vi "deleteBlankData.vi"(8 "error in (no error)":errorcluster, 11 "reference in":refnum<class "Notification Controller.lvclass">) -> (0 "error out":errorcluster, 3 "reference out":refnum<class "Notification Controller.lvclass">)   [LabVIEW 2015, in "Notification Controller.lvclass"]
uses:
  Notification Controller.lvclass
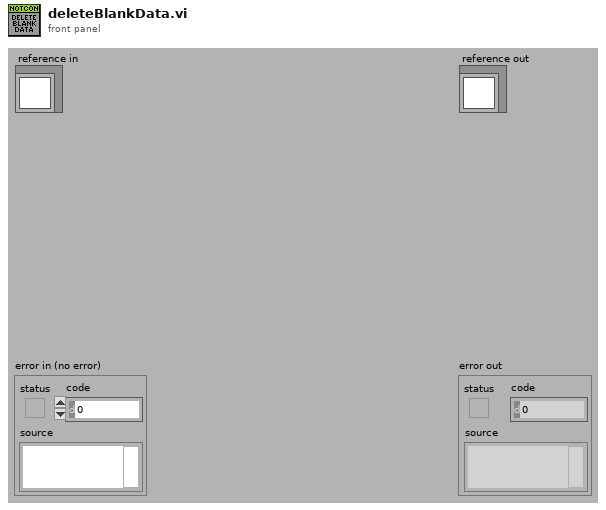
[diagram p1: front panel]
types:
  T1 = typedef "Notification Controller.lvclass/ObjectAttributesRef.ctl" = refnum<data-value>
  T2 = typedef "Notification Controller.lvclass/ObjectAttributes.ctl" = cluster{"MyAttribute":dbl, "items_data":string[][][], "items_notification_refs":refnum<class "itemsNotification.lvclass">[], "notifications_data_items":string[][], "items_nots?":bool, "devices_controller_ref":refnum<class "Devices Controller.lvclass">, "onlineUpdate":timestamp, "notController?":bool, "tracking_notification_ref":refnum<class "trackingNotification.lvclass">, "notifications_data_tracking":string[][], "tracking_parts_data":string[][], "tracking_nots?":bool, "index_tracking_not":i32[], "file_controller_ref":refnum<class "File Controller.lvclass">}
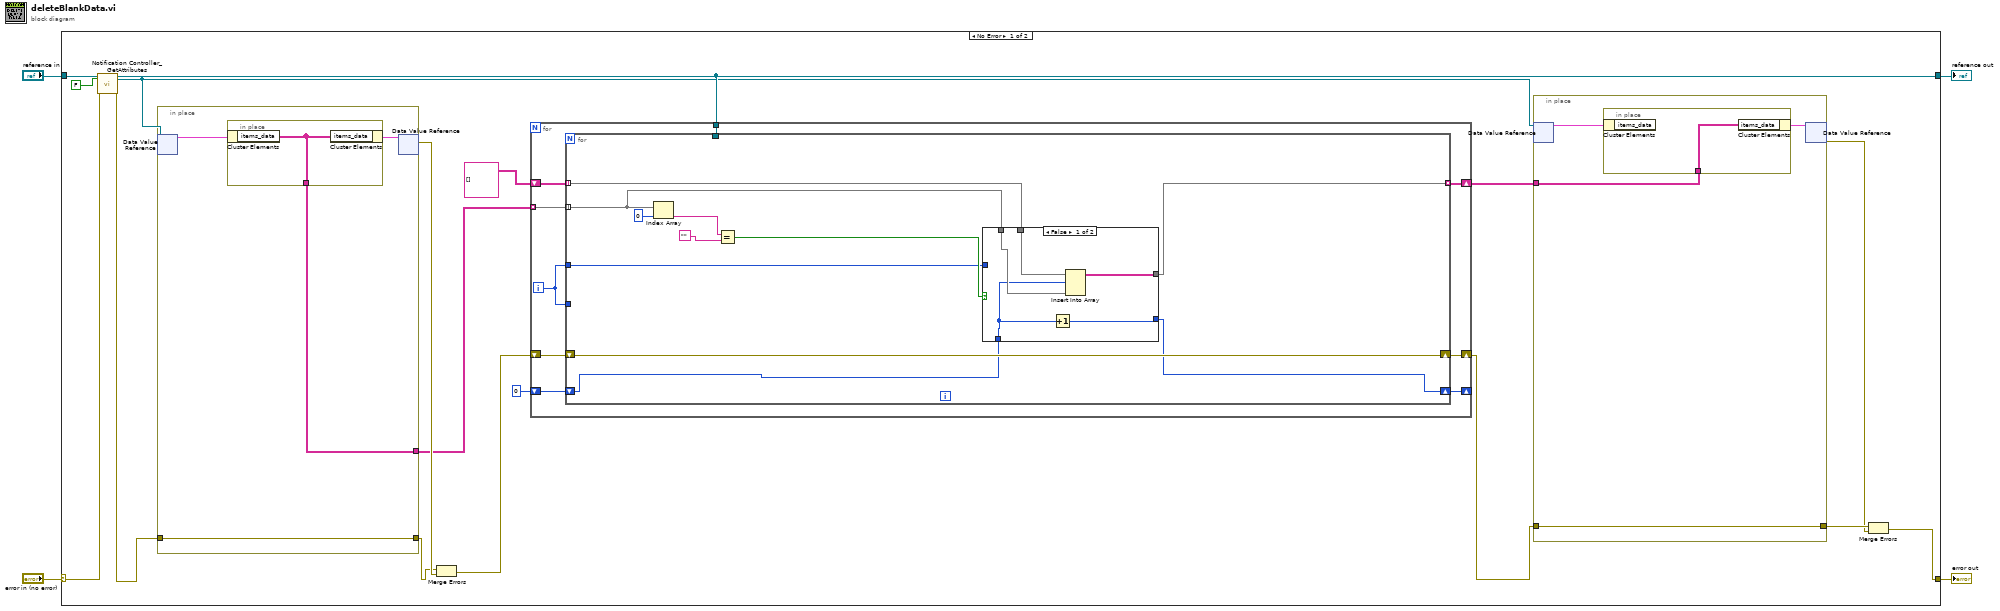
[diagram p0: block diagram]
diagram:
  n1 = case shown="No Error" "error in (no error)" {
    selector: "error in (no error)" -> [w17 w60]
    tunnel: [w7 w60] -> w3
    tunnel: [w12 w59] -> w1
    tunnel: "reference in" -> [w19 w59]
    frame No Error {
      n2 = call "Notification Controller_GetAttributes.vi"("reference in"=w19, "return data? (T)"=FALSE, "error in (no error)"=w17) -> ("reference out"=w12:refnum<class "Notification Controller.lvclass">, "attributes ref"=w10:T1, "error out"=w16:errorcluster)  [unwired: 13 in, 1 out]
      n3 = in-place {
        in-place-border: w16 -> [w55]
        in-place-border: [w55] -> w20
        in-place-border: [w54] -> w14
        n4 = in-place-dvr #1(w10) -> (w56:T2)  [unwired: 1 out]
        n5 = in-place {
          in-place-border: [w58] -> w54
          n6 = in-place-cluster #2(w56) -> ("items_data"=w58:string[][][])
          n7 = in-place-cluster #2("items_data"=w58) -> (w57:T2)
        }
        n8 = in-place-dvr #1(w57) -> (w21:errorcluster)  [unwired: 1 out]
      }
      n9 = Merge Errors(w20, w21) -> (w13:errorcluster)
      n10 = for {
        tunnel: w14 -> [w35] mode=indexing
        shift-right: [w32] -> w11
        shift-left: w13 -> [w34]
        tunnel: w12 -> [w31]
        shift-right: [w29] -> w5
        shift-left: string[][][] [] ("data") -> [w30]
        shift-right: [w27] -> _
        shift-left: 0 -> [w28]
        i -> [w33]
        n11 = for {
          tunnel: w35 -> [w46] mode=indexing
          tunnel: w33 -> [w36]
          tunnel: w33 -> [_]
          shift-right: [w45] -> w32
          shift-left: w34 -> [w45]
          tunnel: w31 -> [_]
          shift-right: [w41] -> w27
          shift-left: w28 -> [w42]
          tunnel: w30 -> [w44] mode=indexing
          tunnel: [w43] -> w29 mode=indexing
          n12 = Index Array(array=w46, index=0) -> (element=w39:string)
          n13 = Equal?(x=w39, y="") -> (x = y?=w37:bool)
          n14 = case shown="False" w37 {
            tunnel: w44 -> [w51 w53]
            tunnel: w46 -> [w48 _]
            tunnel: [w50 w53] -> w43
            tunnel: w42 -> [w47 w52]
            tunnel: [w49 w52] -> w41
            tunnel: w36 -> [_ _]
            frame False {
              n15 = Increment(x=w47) -> (x+1=w49:i32)
              n16 = Insert Into Array(array=w51, index (row)=w47, new element=w48) -> (w50:string[][])  [unwired: 1 in]
            }
            frame True {
            }
          }
        }
      }
      n17 = in-place {
        in-place-border: w11 -> [w23]
        in-place-border: [w23] -> w9
        in-place-border: w5 -> [w22]
        n18 = in-place-dvr #3(w10) -> (w24:T2)  [unwired: 1 out]
        n19 = in-place {
          in-place-border: w22 -> [w26]
          n20 = in-place-cluster #4(w24) -> ()  [unwired: 1 out]
          n21 = in-place-cluster #4("items_data"=w26) -> (w25:T2)
        }
        n22 = in-place-dvr #3(w25) -> (w8:errorcluster)  [unwired: 1 out]
      }
      n23 = Merge Errors(w9, w8) -> (w7:errorcluster)
    }
    frame Error {
    }
  }
  "error out" <- w3
  "reference out" <- w1
